vi "Change_Filename.vi"(8 "error in (no error)":errorcluster, 10 "Filename in":string, 11 "AB_Dest_LLB in":refnum<class "AB_Dest_LLB.lvclass">) -> (0 "error out":errorcluster, 2 "Filename out":string, 3 "AB_Dest_LLB out":refnum<class "AB_Dest_LLB.lvclass">)   [LabVIEW 2020, in "AB_Dest_LLB.lvclass"]
uses:
  <vilib>/AppBuilder/AB_Classes/Destination/Dest_LLB/AB_Dest_LLB.lvclass
  e:/builds/penguin/labview/branches/2020/dev/dist/vi.lib/AppBuilder/AB_Classes/Destination/AB_Destination.lvclass
  <vilib>/AppBuilder/AB_Classes/Destination/AB_Destination.lvclass
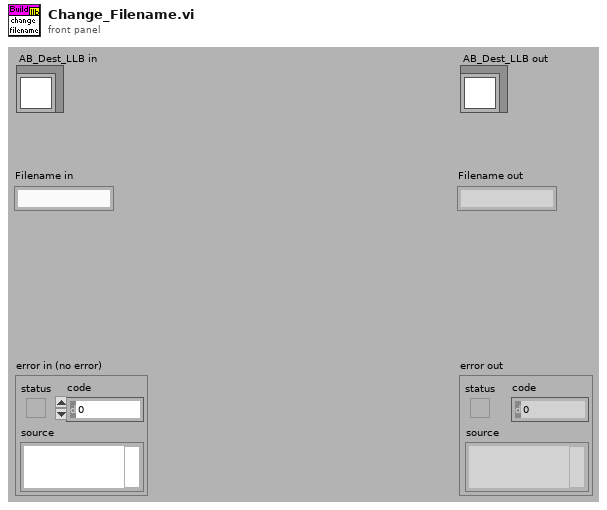
[diagram p1: front panel]
types:
  T1 = typedef "AB_Destination.ctl" = cluster{"destName":string, "path":path, "libraryName":string, "preserveHierarchy":bool, "eng_inBuild":bool, "eng_libraryReference":refnum<vi>, "eng_restictAddToNewLibrary":bool}
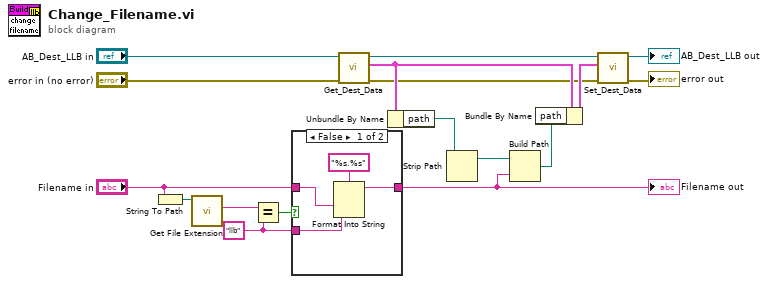
[diagram p0: block diagram]
diagram:
  w16 = "llb" ("y")
  n1 = String To Path(string="Filename in") -> (path=w12:path)
  n2 = call <vilib>:"Get File Extension.vi"("file"=w12) -> ("lowercase file extension"=w11:string)  [unwired: 6 in, 4 out]
  n3 = Equal?(x=w11, y=w16) -> (x = y?=w17:bool)
  n4 = case shown="False" w17 {
    tunnel: [w19 w22] -> w14
    tunnel: "Filename in" -> [w20 w22]
    tunnel: w16 -> [w18 _]
    frame False {
      n5 = Format Into String(format string="%s.%s", w20, w18) -> (resulting string=w19:string)  [unwired: 2 in, 1 out]
    }
    frame True {
    }
  }
  "Filename out" <- w14
  n6 = call <vilib>:"Get_Dest_Data.vi"("error in (no error)"="error in (no error)", "Class in"="AB_Dest_LLB in") -> ("error out"=w4:errorcluster, "destName"=w9:T1, "Class out"=w10:refnum<class "AB_Dest_LLB.lvclass">)  [unwired: 7 in]
  n7 = Unbundle By Name(w9) -> ("path"=w2:path)
  n8 = Strip Path(path=w2) -> (stripped path=w15:path)  [unwired: 1 out]
  n9 = Build Path(base path=w15, name or relative path=w14) -> (appended path=w1:path)
  n10 = Bundle By Name(cluster=w9, "path"=w1) -> (w8:T1)
  n11 = call <vilib>:"Set_Dest_Data.vi"("error in (no error)"=w4, "destName"=w8, "Class in"=w10) -> ("error out"=→"error out":errorcluster, "Class out"=→"AB_Dest_LLB out":refnum<class "AB_Dest_LLB.lvclass">)  [unwired: 7 in]
